vi "Chart[Template].Pause.vi"(8 "error in (no error)":errorcluster, 11 "DisplayWaveforms":refnum<class "DisplayWaveforms.lvclass">) -> (0 "error out":errorcluster, 3 "DisplayWaveforms out":refnum<class "DisplayWaveforms.lvclass">)   [LabVIEW 2020]
doc: "Pause charts"
uses:
  DisplayWaveforms.lvclass
  C:/Program Files (x86)/National Instruments/LabVIEW 2020/vi.lib/JKI/JKI SMO/SMO.UI/SMO.UI.lvclass
  C:/Program Files (x86)/National Instruments/LabVIEW 2020/vi.lib/JKI/JKI SMO/SMO/SMO.lvclass
  C:/Users/mbrij/Dropbox (MIT)/MIT/Research/ASML/Reticle levitation/6dof/Code/LevitationCode/PC/Components/DisplayWaveform/DisplayWaveforms/DisplayWaveforms.lvclass
panel:
  # "For instructions on how to use the JKI State Machine Objects, examples and video tutorials, visit:\nhttp://jki.net/state-machine-objects/\n\nJKI State Machine Objects™\nhttp://jki.net/state-machine-objects/\nCopyright (C) 2005-2015, JKI <info@jki.net>\nALL RIGHTS RESERVED"
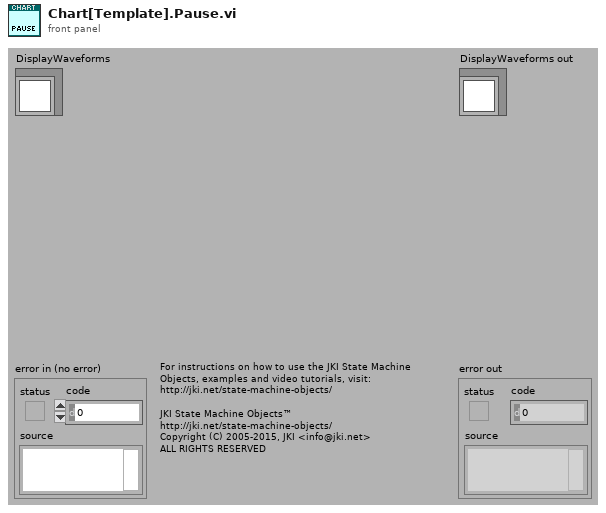
[diagram p1: front panel]
types:
  T1 = typedef "DisplayWaveform.lvlib/DisplayWaveforms.lvclass/PublicEvents--Cluster.ctl" = cluster{"Chart Cleared":refnum<user-event>, "Chart Paused":refnum<user-event>}
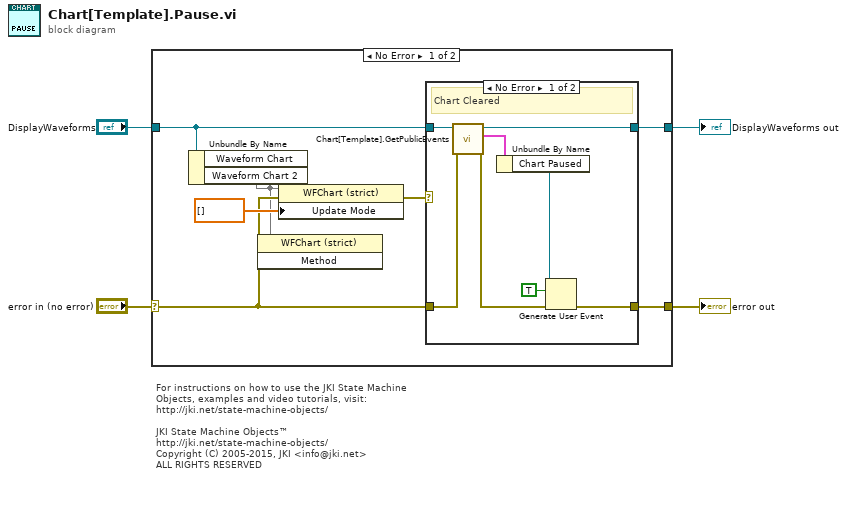
[diagram p0: block diagram]
diagram:
  # "For instructions on how to use the JKI State Machine Objects, examples and video tutorials, visit:\nhttp://jki.net/state-machine-objects/\n\nJKI State Machine Objects™\nhttp://jki.net/state-machine-objects/\nCopyright (C) 2005-2015, JKI <info@jki.net>\nALL RIGHTS RESERVED"
  n1 = case shown="No Error" "error in (no error)" {
    selector: "error in (no error)" -> [w6 w22]
    tunnel: "DisplayWaveforms" -> [w9 w23]
    tunnel: [w11 w22] -> w3
    tunnel: [w10 w23] -> w2
    frame No Error {
      n2 = Unbundle By Name(w9) -> ("Waveform Chart"=w5)  [unwired: 1 out]
      n3 = invoke class="WFChart (strict)" method=#-1(reference=w5) -> ()  [unwired: 2 in, 3 out]
      n4 = property class="WFChart (strict)"(reference=w5, error in=w6, "Update Mode"=dbl[] [] ("History Data")) -> (error out=w7:errorcluster)  [unwired: 1 out]
      n5 = case shown="No Error" w7 {
        tunnel: w6 -> [w17 w20]
        tunnel: [w14 w20] -> w11
        tunnel: w9 -> [w19 w21]
        tunnel: [w18 w21] -> w10
        frame No Error {
          # "Chart Cleared"
          n6 = call "Chart[Template].GetPublicEvents.vi"("error in (no error)"=w17, "DisplayWaveforms"=w19) -> ("error out"=w15:errorcluster, "Chart[Template] Public Events"=w16:T1, "DisplayWaveforms out"=w18:refnum<class "DisplayWaveforms.lvclass">)  [unwired: 7 in]
          n7 = Unbundle By Name(w16) -> ("Chart Paused"=w12:refnum<user-event>)
          n8 = Generate User Event(user event=w12, event data cluster=TRUE ("event data"), error in=w15) -> (error out=w14:errorcluster)  [unwired: 1 in, 1 out]
        }
        frame Error {
          # "Chart was not cleared"
        }
      }
    }
    frame Error {
    }
  }
  "error out" <- w3
  "DisplayWaveforms out" <- w2
